vi "EAGLE RT Illunination Control.vi"(10 "Data":variant, 11 "FPGA Reference":T1) -> (0 "error out":errorcluster)   [LabVIEW 2015]
uses:
  Eagle RT FPGA Ref.ctl
  Controls/Illumination_Control_Struct.ctl
  <vilib>/Utility/error.llb/Error Cluster From Error Code.vi
  <vilib>/rvi/errors/niLvFpgaAdjustHostInterfaceError.vi
  <vilib>/rvi/interface/nirviReadWriteControl/nirviReadWriteControl.xnode
  NiFpgaLv.dll
  <vilib>/rvi/interface/Simulation/niFpgaSimulationCallBeginRW.vi
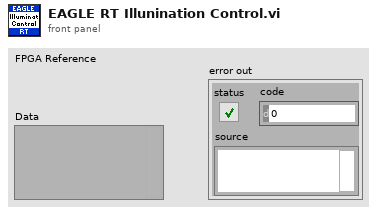
[diagram p1: front panel]
types:
  T1 = typedef "Eagle RT FPGA Ref.ctl" = refnum<k20>
  T2 = typedef "Illumination_Control_Struct.ctl" = cluster{"HRange_Level":dbl, "HRange_OnOff":bool, "VRange_Level":dbl, "VRange_OnOff":bool, "Aim_Level":dbl, "Aim_OnOff":bool, "LED Ring_Level":dbl, "LEDRing_OnOff":bool, "RedDots_Level":dbl, "RedDots_State":enum16{"Off", "Right", "Left"}, "Master Enable":bool}
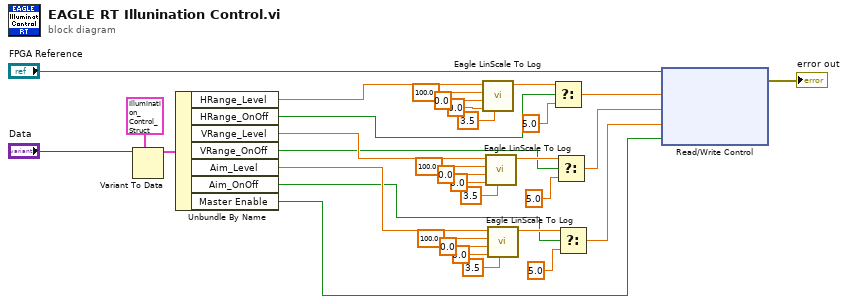
[diagram p0: block diagram]
diagram:
  n1 = Variant To Data(type=T2 {"HRange_Level"=0.0, "HRange_OnOff"=FALSE, "VRange_Level"=0.0, "VRange_OnOff"=FALSE, "Aim_Level"=0.0, "Aim_OnOff"=FALSE, "LED Ring_Level"=0.0, "LEDRing_OnOff"=FALSE, "RedDots_Level"=0.0, "RedDots_State"=enum."Off", "Master Enable"=FALSE} ("Illumination_Ctrl"), Variant="Data") -> (data=w11:T2)  [unwired: 1 in, 1 out]
  n2 = Unbundle By Name(w11) -> ("HRange_Level"=w8:dbl, "HRange_OnOff"=w7:bool, "VRange_Level"=w6:dbl, "VRange_OnOff"=w5:bool, "Aim_Level"=w4:dbl, "Aim_OnOff"=w3:bool, "Master Enable"=w1:bool)
  n3 = call "Eagle LinScale To Log.vi"("MinScaleOut"=3.5, "MaxScaleOut"=0.0, "MinScaleIn"=0.0, "MaxScaleIn"=100.0, "ValIn"=w8) -> ("ValOut"=w16:dbl)  [unwired: 6 in]
  n4 = call "Eagle LinScale To Log.vi"("MinScaleOut"=3.5, "MaxScaleOut"=0.0, "MinScaleIn"=0.0, "MaxScaleIn"=100.0, "ValIn"=w6) -> ("ValOut"=w19:dbl)  [unwired: 6 in]
  n5 = call "Eagle LinScale To Log.vi"("MinScaleOut"=3.5, "MaxScaleOut"=0.0, "MinScaleIn"=0.0, "MaxScaleIn"=100.0, "ValIn"=w4) -> ("ValOut"=w28:dbl)  [unwired: 6 in]
  n6 = Select(t=w16, s=w7, f=5.0) -> (s? t:f=w31:dbl)
  n7 = Select(t=w19, s=w5, f=5.0) -> (s? t:f=w32:dbl)
  n8 = Select(t=w28, s=w3, f=5.0) -> (s? t:f=w33:dbl)
  n9 = xnode "Read/Write Control"("FPGA VI Reference In"="FPGA Reference", "H Range Ctrl"=w31, "V Range Ctrl"=w32, "Aim Ctrl"=w33, "Illumination_Ena"=w1) -> ("error out"=→"error out":errorcluster)  [unwired: 1 in, 1 out]
